vi "AutoClimbNavX.vi"(8 "Stage":i8, 9 "Elevator Encoder":i32, 10 "Horse Encoder":i32) -> (1 "Elevator Output":dbl, 2 "Horse Output":dbl)   [LabVIEW 2018]
uses:
  <vilib>/addons/control/pid/pid.llb/PID (DBL).vi
  <vilib>/addons/control/pid/NI_PID_pid.lvlib
panel:
  in  "Elevator PID Gains":T1={"proportional gain (Kc)"=1e-06, "integral time (Ti, min)"=0.0, "derivative time (Td, min)"=0.0}
  in  "Horse PID Gains":T1={"proportional gain (Kc)"=-1e-05, "integral time (Ti, min)"=0.0, "derivative time (Td, min)"=0.0}
  in  "Elevator Setpoint":i32
  in  "Horse Setpoint":i32=-180000
  in  "Elevator Gyro P Val":dbl=10.0
  in  "Horse Gyro P Val":dbl=-10.0
  out "Gyro Values":T2
  # "Horse: Neg P gyro val\nElevator: Pos gyro val\n\nHorse: Pos gain\nElevator: Pos gain"
  # "Neg"
  # "Pos"
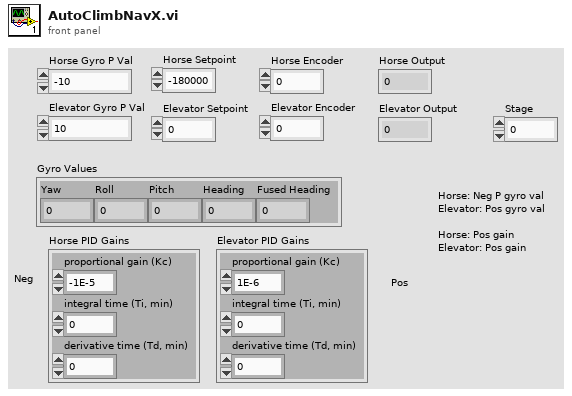
[diagram p1: front panel]
types:
  T1 = cluster{"proportional gain (Kc)":dbl, "integral time (Ti, min)":dbl, "derivative time (Td, min)":dbl}
  T2 = cluster{"Yaw":dbl, "Roll":dbl, "Pitch":dbl, "Heading":dbl, "Fused Heading":dbl}
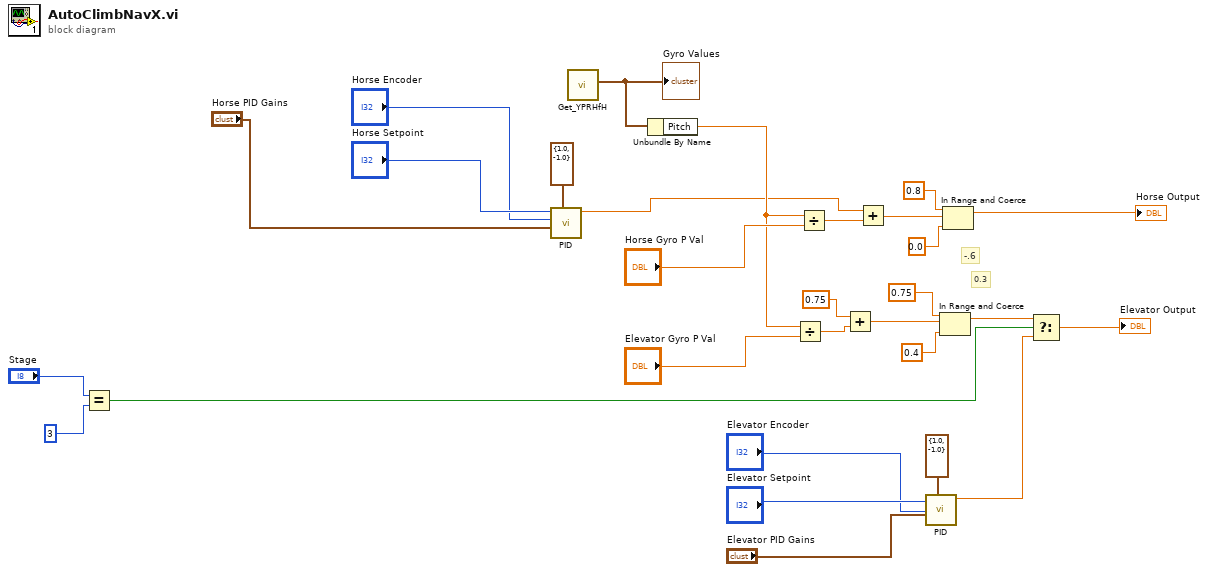
[diagram p0: block diagram]
diagram:
  # "0.3"
  # "-.6"
  n1 = Equal?(x="Stage", y=i8 3) -> (x = y?=w3:bool)
  n2 = call-poly <vilib>:"PID.vi"("output range"=cluster{"output high":dbl, "output low":dbl} {"output high"=1.0, "output low"=-1.0}, "PID gains"="Horse PID Gains", "process variable"="Horse Encoder", "setpoint"="Horse Setpoint") -> ("output"=w15:dbl)  [unwired: 6 in, 1 out]
  n3 = call <vilib>:"Get_YPRHfH.vi"() -> ("YRPHfH"=w29:T2)  [unwired: 11 in]
  "Gyro Values" <- w29
  n4 = Unbundle By Name(w29) -> ("Pitch"=w21:dbl)
  n5 = Divide(x=w21, y="Elevator Gyro P Val") -> (x/y=w18:dbl)
  n6 = Divide(x=w21, y="Horse Gyro P Val") -> (x/y=w19:dbl)
  n7 = Add(x=0.75, y=w18) -> (x+y=w17:dbl)
  n8 = Add(x=w15, y=w19) -> (x+y=w20:dbl)
  n9 = call-poly <vilib>:"PID.vi"("output range"=cluster{"output high":dbl, "output low":dbl} {"output high"=1.0, "output low"=-1.0}, "PID gains"="Elevator PID Gains", "process variable"="Elevator Encoder", "setpoint"="Elevator Setpoint") -> ("output"=w6:dbl)  [unwired: 6 in, 1 out]
  n10 = In Range and Coerce(upper limit=0.75, x=w17, lower limit=0.4) -> (coerced(x)=w5:dbl)  [unwired: 1 out]
  n11 = In Range and Coerce(upper limit=0.8, x=w20, lower limit=0.0) -> (coerced(x)=→"Horse Output":dbl)  [unwired: 1 out]
  n12 = Select(t=w5, s=w3, f=w6) -> (s? t:f=→"Elevator Output":dbl)
